vi "Test Valid Path to File.vi"(11 "Test Case In":refnum<class "Test File Exists.lvclass">) -> (0 "error out":errorcluster, 3 "Test Case Out":refnum<class "Test File Exists.lvclass">)   [LabVIEW 2024, in "Test File Exists.lvclass"]
uses:
  Test File Exists.lvclass
  C:/Program Files/National Instruments/LabVIEW 2025/vi.lib/Astemes/LUnit/Test Case.lvclass
  <vilib>/Astemes/LUnit/Test Case.lvclass/Test Case.ctl
  Source/Common Helpers.lvlib
  <vilib>/Astemes/LUnit/Test Case.lvclass
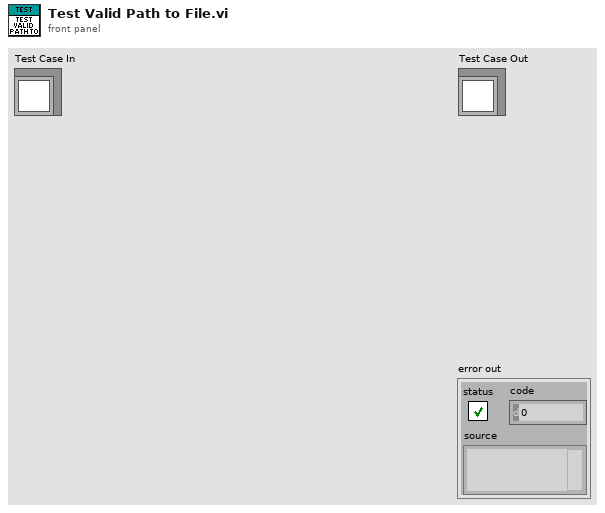
[diagram p1: front panel]
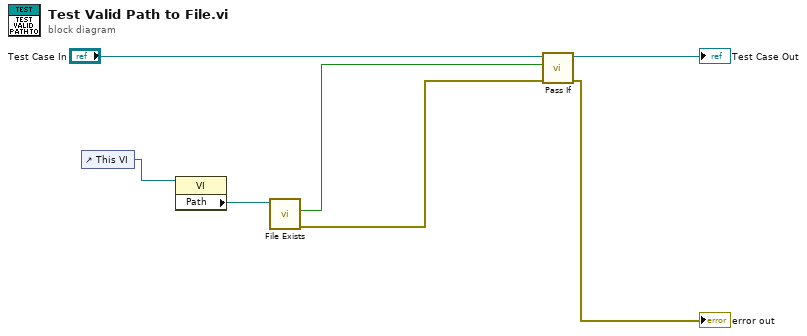
[diagram p0: block diagram]
diagram:
  n1 = control-ref of="This VI"() -> (w4:refnum<vi>)
  n2 = property class="VI"(reference=w4) -> ("Path"=w3:path)  [unwired: 1 in, 2 out]
  n3 = call "File Exists.vi"("File Path"=w3) -> ("error out"=w2:errorcluster, "Exists"=w1:bool)  [unwired: 8 in, 1 out]
  n4 = call <vilib>:"Pass If.vi"("error in (no error)"=w2, "Pass?"=w1, "LUnit Test Case In"="Test Case In") -> ("error out"=→"error out":errorcluster, "LUnit Test Case Out"=→"Test Case Out":refnum<class "Test File Exists.lvclass">)  [unwired: 7 in]
